vi "Add pass.vi"(0 "vi path":path) -> ()   [LabVIEW 2015]
panel:
  in  "Case Constant\n(See Context Help) 2":bool
  in  "Case Constant\n(See Context Help)":bool
  out "Contents":string[][](array[string])
  in  "Exit":bool
  in  "ADD":bool
  in  "Password":string
  in  "User Name":string
  in  "Group":u16(ring) items=["admin", "user"]
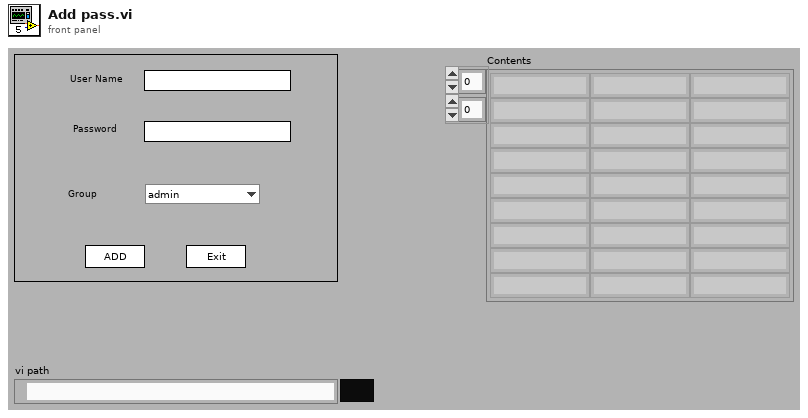
[diagram p1: front panel]
types:
  T1 = enum16{"open", "open or create", "create or replace", "create", "open (read only)"}
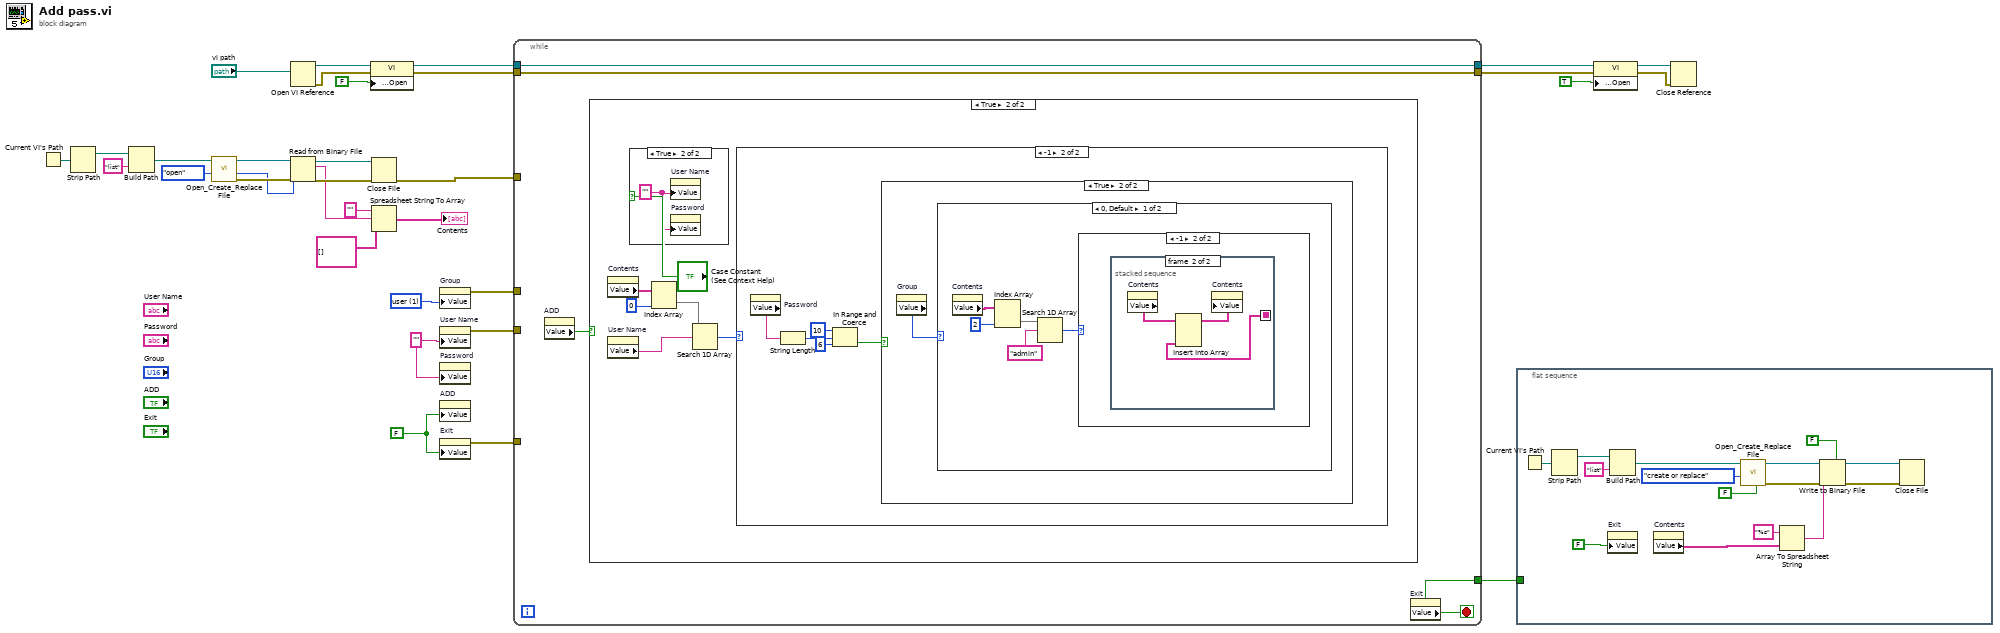
[diagram p0: block diagram]
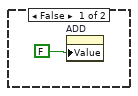
[diagram p2: hidden frame]
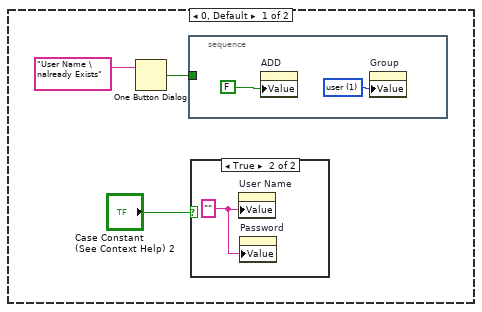
[diagram p4: hidden frame]
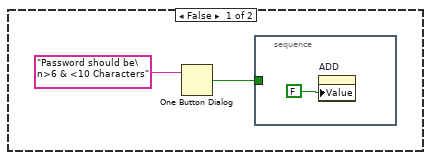
[diagram p6: hidden frame]
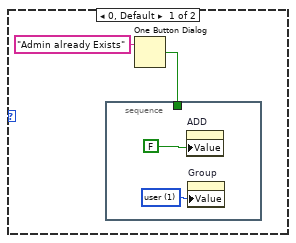
[diagram p7: hidden frame]
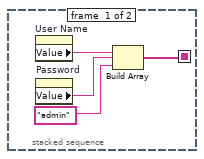
[diagram p8: hidden frame]
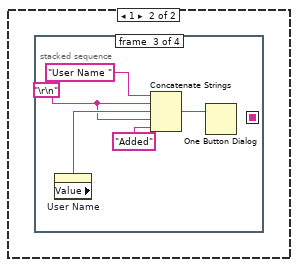
[diagram p9: hidden frame]
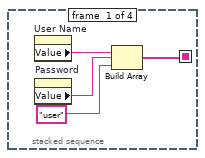
[diagram p10: hidden frame]
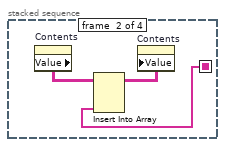
[diagram p11: hidden frame]
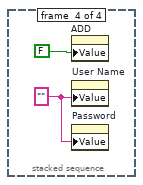
[diagram p12: hidden frame]
diagram:
  w19 = u16 1 items=["admin", "user"] ("Group")
  w22 = FALSE ("ADD")
  w12 = "" ("User Name")
  n1 = Current VI's Path() -> (path=w4:path)
  n2 = Strip Path(path=w4) -> (stripped path=w3:path)  [unwired: 1 out]
  n3 = Build Path(base path=w3, name or relative path="list") -> (appended path=w1:path)
  n4 = call <vilib>:"Open_Create_Replace File.vi"("function (open:0)"=T1."open", "file path"=w1) -> ("error out"=w33:errorcluster, "file size (bytes)"=w29:i32, "refnum"=w32:refnum<file>)  [unwired: 6 in, 1 out]
  n5 = Open VI Reference(vi path="vi path") -> (vi reference=w16:refnum<vi>, error out=w10:errorcluster)  [unwired: 5 in]
  n6 = Read from Binary File(8:w33, 10:w29, 11:w32) -> (0:w31:errorcluster, 2:w28:string, 3:w30:refnum<file>)  [unwired: 3 in, 1 out]
  n7 = property class="VI"(reference=w16, error in=w10, "Front Panel Window:Open"=FALSE) -> (reference out=w15:refnum<vi>, error out=w14:errorcluster)
  n8 = Close File(refnum=w30, error in=w31) -> (error out=w24:errorcluster)  [unwired: 1 out]
  n9 = Spreadsheet String To Array(format string="", spreadsheet string=w28, array type (2D Dbl)=string[][] []) -> (array=→"Contents":string[][])  [unwired: 1 in]
  n10 = property on="Group" class="Ring (strict)"("Value"=w19) -> (error out=w18:errorcluster)  [unwired: 2 in, 1 out]
  n11 = property on="User Name" class="Str"("Value"=w12) -> (error out=w23:errorcluster)  [unwired: 2 in, 1 out]
  n12 = property on="Password" class="Str"("Value"=w12) -> ()  [unwired: 2 in, 2 out]
  n13 = property on="ADD" class="Bool (strict)"("Value"=w22) -> ()  [unwired: 2 in, 2 out]
  n14 = property on="Exit" class="Bool (strict)"("Value"=w22) -> (error out=w21:errorcluster)  [unwired: 2 in, 1 out]
  n15 = while {
    tunnel: w24 -> [_]
    tunnel: w23 -> [_]
    tunnel: w21 -> [_]
    tunnel: [w34] -> w20
    tunnel: w18 -> [_]
    tunnel: w15 -> [w36]
    tunnel: w14 -> [w35]
    tunnel: [w36] -> w8
    tunnel: [w35] -> w7
    stop <- w34 stop-if-true
    n16 = property on="ADD" class="Bool (strict)"() -> ("Value"=w37:bool)  [unwired: 2 in, 2 out]
    n17 = case shown="True" w37 {
      frame False {
        n18 = property on="ADD" class="Bool (strict)"("Value"=FALSE ("ADD")) -> ()  [unwired: 2 in, 2 out]
      }
      frame True {
        n19 = property on="Contents" class="Arr (strict)"() -> ("Value"=w44:string[][])  [unwired: 2 in, 2 out]
        n20 = property on="User Name" class="Str"() -> ("Value"=w42:string)  [unwired: 2 in, 2 out]
        n21 = case shown="True" "Case Constant\n(See Context Help)" {
          frame False {
          }
          frame True {
            w45 = "" ("User Name")
            n22 = property on="User Name" class="Str"("Value"=w45) -> ()  [unwired: 2 in, 2 out]
            n23 = property on="Password" class="Str"("Value"=w45) -> ()  [unwired: 2 in, 2 out]
          }
        }
        n24 = Index Array(array=w44, index (col)=0 ("disabled index (col)")) -> (element=w40:string[])  [unwired: 1 in]
        n25 = Search 1D Array(1D array=w40, element=w42) -> (index of element=w41:i32)  [unwired: 1 in]
        n26 = case shown="-1" w41 {
          frame 0, Default {
            n27 = One Button Dialog(message="User Name \nalready Exists") -> (true=w47:bool)  [unwired: 1 in]
            n28 = stacked-sequence {
              tunnel: w47 -> [_]
              frame #0 {
                w50 = u16 1 items=["admin", "user"] ("Group")
                n29 = property on="ADD" class="Bool (strict)"("Value"=FALSE ("ADD")) -> ()  [unwired: 2 in, 2 out]
                n30 = property on="Group" class="Ring (strict)"("Value"=w50) -> ()  [unwired: 2 in, 2 out]
              }
            }
            n31 = case shown="True" "Case Constant\n(See Context Help) 2" {
              frame False {
              }
              frame True {
                w49 = "" ("User Name")
                n32 = property on="User Name" class="Str"("Value"=w49) -> ()  [unwired: 2 in, 2 out]
                n33 = property on="Password" class="Str"("Value"=w49) -> ()  [unwired: 2 in, 2 out]
              }
            }
          }
          frame -1 {
            n34 = property on="Password" class="Str"() -> ("Value"=w52:string)  [unwired: 2 in, 2 out]
            n35 = String Length(string=w52) -> (length=w56:i32)
            n36 = In Range and Coerce(upper limit=10, x=w56, lower limit=6) -> (In Range?=w53:bool)  [unwired: 1 out]
            n37 = case shown="True" w53 {
              frame False {
                n38 = One Button Dialog(message="Password should be\n>6 & <10 Characters") -> (true=w57:bool)  [unwired: 1 in]
                n39 = stacked-sequence {
                  tunnel: w57 -> [_]
                  frame #0 {
                    n40 = property on="ADD" class="Bool (strict)"("Value"=FALSE ("ADD")) -> ()  [unwired: 2 in, 2 out]
                  }
                }
              }
              frame True {
                n41 = property on="Group" class="Ring (strict)"() -> ("Value"=w60:u16)  [unwired: 2 in, 2 out]
                n42 = case shown="0, Default" w60 {
                  frame 0, Default {
                    n43 = property on="Contents" class="Arr (strict)"() -> ("Value"=w64:string[][])  [unwired: 2 in, 2 out]
                    n44 = Index Array(array=w64, index (col)=2 ("disabled index (col)")) -> (element=w63:string[])  [unwired: 1 in]
                    n45 = Search 1D Array(1D array=w63, element="admin") -> (index of element=w61:i32)  [unwired: 1 in]
                    n46 = case shown="-1" w61 {
                      frame 0, Default {
                        n47 = One Button Dialog(message="Admin already Exists") -> (true=w66:bool)  [unwired: 1 in]
                        n48 = stacked-sequence {
                          tunnel: w66 -> [_]
                          frame #0 {
                            w68 = u16 1 items=["admin", "user"] ("Group")
                            n49 = property on="ADD" class="Bool (strict)"("Value"=FALSE ("ADD")) -> ()  [unwired: 2 in, 2 out]
                            n50 = property on="Group" class="Ring (strict)"("Value"=w68) -> ()  [unwired: 2 in, 2 out]
                          }
                        }
                      }
                      frame -1 {
                        n51 = stacked-sequence {
                          seq-local: [w70 _] -> [_ w74]
                          frame #0 {
                            n52 = property on="User Name" class="Str"() -> ("Value"=w73:string)  [unwired: 2 in, 2 out]
                            n53 = property on="Password" class="Str"() -> ("Value"=w72:string)  [unwired: 2 in, 2 out]
                            n54 = Build Array(w73, w72, "admin") -> (w70:string[])
                          }
                          frame #1 {
                            n55 = property on="Contents" class="Arr (strict)"() -> ("Value"=w76:string[][])  [unwired: 2 in, 2 out]
                            n56 = Insert Into Array(array=w76, new element=w74) -> (w75:string[][])  [unwired: 2 in]
                            n57 = property on="Contents" class="Arr (strict)"("Value"=w75) -> ()  [unwired: 2 in, 2 out]
                          }
                        }
                      }
                    }
                  }
                  frame 1 {
                    n58 = stacked-sequence {
                      seq-local: [w78 _ _ _] -> [_ w81 _ _]
                      frame #0 {
                        n59 = property on="User Name" class="Str"() -> ("Value"=w80:string)  [unwired: 2 in, 2 out]
                        n60 = property on="Password" class="Str"() -> ("Value"=w79:string)  [unwired: 2 in, 2 out]
                        n61 = Build Array(w80, w79, "user") -> (w78:string[])
                      }
                      frame #1 {
                        n62 = property on="Contents" class="Arr (strict)"() -> ("Value"=w83:string[][])  [unwired: 2 in, 2 out]
                        n63 = Insert Into Array(array=w83, new element=w81) -> (w82:string[][])  [unwired: 2 in]
                        n64 = property on="Contents" class="Arr (strict)"("Value"=w82) -> ()  [unwired: 2 in, 2 out]
                      }
                      frame #2 {
                        w85 = "\r\n"
                        n65 = property on="User Name" class="Str"() -> ("Value"=w86:string)  [unwired: 2 in, 2 out]
                        n66 = Concatenate Strings("User Name " ("string"), w85, w86, w85, "Added" ("string")) -> (w88:string)
                        n67 = One Button Dialog(message=w88) -> ()  [unwired: 1 in, 1 out]
                      }
                      frame #3 {
                        w89 = "" ("User Name")
                        n68 = property on="ADD" class="Bool (strict)"("Value"=FALSE ("ADD")) -> ()  [unwired: 2 in, 2 out]
                        n69 = property on="User Name" class="Str"("Value"=w89) -> ()  [unwired: 2 in, 2 out]
                        n70 = property on="Password" class="Str"("Value"=w89) -> ()  [unwired: 2 in, 2 out]
                      }
                    }
                  }
                }
              }
            }
          }
        }
      }
    }
    n71 = property on="Exit" class="Bool (strict)"() -> ("Value"=w34:bool)  [unwired: 2 in, 2 out]
  }
  n72 = flat-sequence {
    tunnel: w20 -> [_]
    frame #0 {
      n73 = Current VI's Path() -> (path=w95:path)
      n74 = Strip Path(path=w95) -> (stripped path=w94:path)  [unwired: 1 out]
      n75 = property on="Exit" class="Bool (strict)"("Value"=FALSE ("ADD")) -> ()  [unwired: 2 in, 2 out]
      n76 = Build Path(base path=w94, name or relative path="list") -> (appended path=w92:path)
      n77 = property on="Contents" class="Arr (strict)"() -> ("Value"=w102:string[][])  [unwired: 2 in, 2 out]
      n78 = call <vilib>:"Open_Create_Replace File.vi"("advisory dialog? (display:T)"=FALSE, "function (open:0)"=T1."create or replace", "file path"=w92) -> ("error out"=w103:errorcluster, "refnum"=w104:refnum<file>)  [unwired: 5 in, 2 out]
      n79 = Array To Spreadsheet String(array=w102, 3:"%s" ("format string")) -> (spreadsheet string=w101:string)  [unwired: 1 in]
      n80 = Write to Binary File(file (use dialog)=w104, data=w101, error in=w103, 5:FALSE ("prepend array or string size? (T)")) -> (refnum out=w96:refnum<file>, error out=w97:errorcluster)  [unwired: 2 in, 1 out]
      n81 = Close File(refnum=w96, error in=w97) -> ()  [unwired: 2 out]
    }
  }
  n82 = property class="VI"(reference=w8, error in=w7, "Front Panel Window:Open"=TRUE) -> (reference out=w6:refnum<vi>, error out=w5:errorcluster)
  n83 = Close Reference(reference=w6, error in (no error)=w5) -> ()  [unwired: 1 out]
